vi "Edit Line.vi"(8 "error in":errorcluster, 10 "Line Name":string, 11 "References":T1) -> (0 "error out":errorcluster, 2 "change?":bool)   [LabVIEW 2018, in "Add Module editor node.lvclass"]
doc: "This VI edits the properties of a line. It will unlink channels and tags and create new links to channels and tags."
uses:
  Add Module editor node.lvclass
  <vilib>/NI/DCAF/Tag Editor Core/Table API/Table Manager/object ref.ctl
  <vilib>/NI/DCAF/Tag Editor Core/Configuration Editor/Classes/Engine Parent/Engine Parent Editor Node.lvclass
  <vilib>/NI/DCAF/Tag Editor Core/Configuration Editor/Classes/Module editor node/module editor node.lvclass
  module/configuration/Add Module configuration.lvclass
  C:/Program Files (x86)/National Instruments/LabVIEW 2018/vi.lib/NI/Configuration Framework/serializable configuration/NISE_CEF_serializable configuration.lvclass
  module/configuration/Add Module configuration.lvclass/Add Module configuration.ctl
  <vilib>/NI/Configuration Framework/serializable configuration/NISE_CEF_serializable configuration.lvclass/NISE_CEF_serializable configuration.ctl
  <vilib>/Utility/LVClass/Get LV Class Name.vi
  <vilib>/NI/Configuration Framework/error generator/NISE_error generator.vi
  <vilib>/NI/Tag Bus Module Framework/channel/TBM channel.lvclass
  <vilib>/NI/Configuration Framework/serializable configuration/NISE_CEF_serializable configuration.lvclass
  <vilib>/NI/DCAF/Tag Editor Core/Table API/Table Manager/Table Manager.lvclass
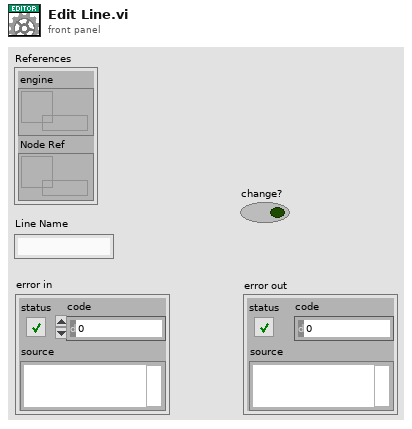
[diagram p1: front panel]
types:
  T1 = typedef "Table Manager.lvlib/Table Manager.lvclass/object ref.ctl" = cluster{"engine":refnum<data-value>, "Node Ref":refnum<data-value>}
  T2 = typedef "Add Module configuration.lvclass/Line.ctl" = cluster{"channel":refnum<class "TBM channel.lvclass">}
  T3 = typedef "Add Module editor node.lvclass/Mappings.ctl" = cluster{"Line":T2, "Maps":T4[]}
  T4 = typedef "Add Module editor node.lvclass/Map.ctl" = cluster{"channel":refnum<class "TBM channel.lvclass">, "tag name":string}
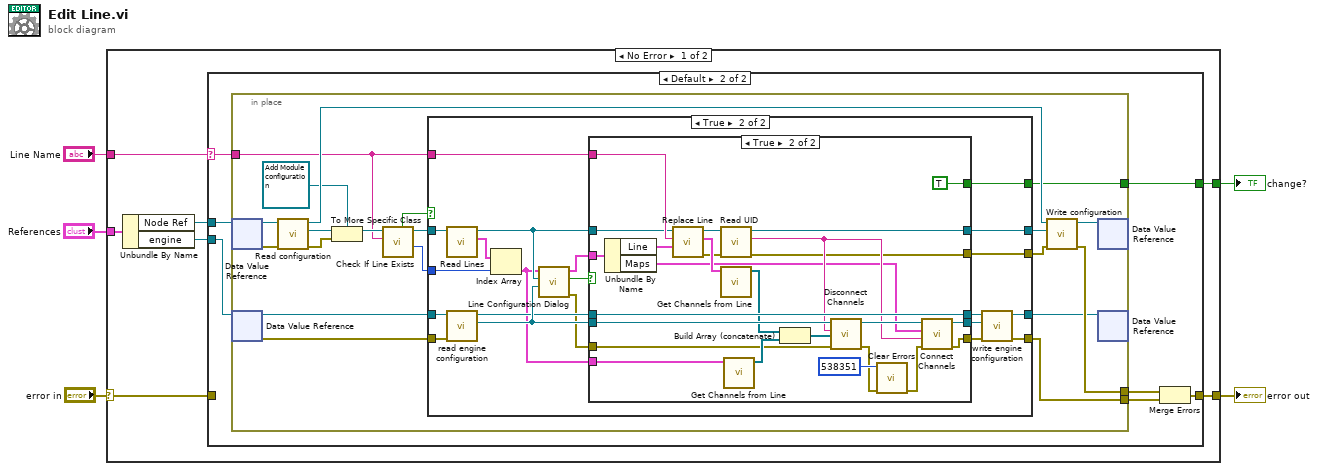
[diagram p0: block diagram]
diagram:
  n1 = case shown="No Error" "error in" {
    selector: "error in" -> [w6 w94]
    tunnel: "References" -> [w10 _]
    tunnel: "Line Name" -> [w7 _]
    tunnel: [w9 w94] -> w2
    tunnel: [w8 _] -> w1
    frame No Error {
      n2 = Unbundle By Name(w10) -> ("Node Ref"=w12:refnum<data-value>, "engine"=w11:refnum<data-value>)
      n3 = case shown="Default" w7 {
        selector: w7 -> [_ w14]
        tunnel: w12 -> [_ w20]
        tunnel: w11 -> [_ w19]
        tunnel: [w13 w16] -> w9
        tunnel: [_ w15] -> w8
        tunnel: w6 -> [w13 _]
        frame " " {
        }
        frame Default {
          n4 = in-place {
            in-place-border: [w28] -> w18
            in-place-border: [w22] -> w17
            in-place-border: [w27] -> w15
            in-place-border: w14 -> [w32]
            n5 = in-place-dvr #1(w20) -> (w39:refnum<class "module editor node.lvclass">, w33:errorcluster)
            n6 = in-place-dvr #2(w19) -> (w25:refnum<class "Engine Parent Editor Node.lvclass">, w24:errorcluster)
            n7 = call-dynamic "Read configuration.vi"("error in"=w33, "NISE_CEF_serializable node in"=w39) -> ("error out"=w36:errorcluster, "configuration"=w37:refnum<class "NISE_CEF_serializable configuration.lvclass">, "NISE_CEF_serializable node out"=w38:refnum<class "module editor node.lvclass">)  [unwired: 7 in]
            n8 = To More Specific Class(target class=refnum<class "Add Module configuration.lvclass"> refnum ("tag bus configurable plugin module configuration"), reference=w37, error in=w36) -> (specific class reference=w34:refnum<class "Add Module configuration.lvclass">)  [unwired: 1 out]
            n9 = call-dynamic "Check If Line Exists.vi"("Name to Locate"=w32, "Add Module configuration in"=w34) -> ("Index"=w29:i32, "Add Module configuration out"=w30:refnum<class "Add Module configuration.lvclass">, "Found?"=w26:bool)  [unwired: 5 in, 2 out]
            n10 = case shown="True" w26 {
              tunnel: w30 -> [w43 w63]
              tunnel: w32 -> [_ w64]
              tunnel: [w43 w58] -> w31
              tunnel: w29 -> [_ w60]
              tunnel: [_ w56] -> w27
              tunnel: w25 -> [w42 w55]
              tunnel: w24 -> [w41 w54]
              tunnel: [w42 w52] -> w23
              tunnel: [w41 w51] -> w22
              tunnel: [_ w44] -> w21
              frame False {
              }
              frame True {
                n11 = call "Read Lines.vi"("Add Module configuration in"=w63) -> ("Lines"=w61:T2[], "Add Module configuration out"=w62:refnum<class "Add Module configuration.lvclass">)  [unwired: 8 in, 1 out]
                n12 = call <vilib>:"read engine configuration.vi"("error in"=w54, "Engine Parent Editor Node in"=w55) -> ("engine configuration"=w53:refnum<class "engine configuration.lvclass">, "Engine Parent Editor Node out"=w49:refnum<class "Engine Parent Editor Node.lvclass">)  [unwired: 7 in, 1 out]
                n13 = Index Array(array=w61, index=w60) -> (element=w45:T2)
                n14 = call "Line Configuration Dialog.vi"("engine configuration in"=w53, "tag bus configurable plugin module configuration"=w62, "Line"=w45) -> ("error out"=w46:errorcluster, "changed"=w57:bool, "Mappings out"=w59:T3)  [unwired: 5 in, 1 out]
                n15 = case shown="True" w57 {
                  tunnel: w64 -> [_ w93]
                  tunnel: w53 -> [w67 w92]
                  tunnel: w62 -> [w68 w89]
                  tunnel: w59 -> [_ w88]
                  tunnel: [w68 w86] -> w58
                  tunnel: [_ TRUE ("change?")] -> w56
                  tunnel: [w67 w83] -> w48
                  tunnel: [w66 w82] -> w50
                  tunnel: w49 -> [w66 w82]
                  tunnel: [w65 w80] -> w47
                  tunnel: w46 -> [w65 w75]
                  tunnel: w45 -> [_ w71]
                  tunnel: [_ w69] -> w44
                  frame False {
                  }
                  frame True {
                    n16 = Unbundle By Name(w88) -> ("Line"=w87:T2, "Maps"=w79:T4[])
                    n17 = call "Replace Line.vi"("New Line"=w87, "Line Name"=w93, "Add Module configuration in"=w89) -> ("error out"=w70:errorcluster, "Old Line"=w90:T2, "Add Module configuration out"=w91:refnum<class "Add Module configuration.lvclass">)  [unwired: 6 in]
                    n18 = call <vilib>:"Read UID.vi"("error in"=w70, "configuration in"=w91) -> ("error out"=w69:errorcluster, "instance id"=w81:string, "configuration out"=w86:refnum<class "Add Module configuration.lvclass">)  [unwired: 7 in]
                    n19 = call "Get Channels from Line.vi"("Line"=w90) -> ("Channels"=w78:refnum<class "TBM channel.lvclass">[])  [unwired: 10 in]
                    n20 = call "Get Channels from Line.vi"("Line"=w71) -> ("Channels"=w77:refnum<class "TBM channel.lvclass">[])  [unwired: 10 in]
                    n21 = Build Array (concatenate)(w78, w77) -> (w76:refnum<class "TBM channel.lvclass">[])
                    n22 = call "Disconnect Channels.vi"("error in (no error)"=w75, "Deleted Channels"=w76, "instance id"=w81, "Engine Configuration in"=w92) -> ("error out"=w73:errorcluster, "Engine Configuration out"=w85:refnum<class "engine configuration.lvclass">)  [unwired: 6 in]
                    n23 = call <vilib>:"Clear Errors.vi"("error in (no error)"=w73, "specific error code to clear (0: all)"=538351) -> ("error out"=w72:errorcluster)  [unwired: 4 in, 1 out]
                    n24 = call "Connect Channels.vi"("error in (no error)"=w72, "instance id"=w81, "Maps"=w79, "Engine Configuration in"=w85) -> ("error out"=w80:errorcluster, "Engine Configuration out"=w83:refnum<class "engine configuration.lvclass">)  [unwired: 6 in]
                  }
                }
                n25 = call <vilib>:"write engine configuration.vi"("error in"=w47, "engine configuration"=w48, "Engine Parent Editor Node in"=w50) -> ("error out"=w51:errorcluster, "Engine Parent Editor Node out"=w52:refnum<class "Engine Parent Editor Node.lvclass">)  [unwired: 7 in]
              }
            }
            n26 = call-dynamic "Write configuration.vi"("error in"=w21, "configuration"=w31, "NISE_CEF_serializable node in"=w38) -> ("error out"=w28:errorcluster, "NISE_CEF_serializable node out"=w40:refnum<class "module editor node.lvclass">)  [unwired: 7 in]
            n27 = in-place-dvr #1(w40) -> ()  [unwired: 2 out]
            n28 = in-place-dvr #2(w23) -> ()  [unwired: 2 out]
          }
          n29 = Merge Errors(w18, w17) -> (w16:errorcluster)
        }
      }
    }
    frame Error {
    }
  }
  "change?" <- w1
  "error out" <- w2
